vi "TSM SSC DAQmx Configure Digital Edge Start trigger PXI Trig.vi"(0 "DAQ TSM in":T1, 5 "source(PXI_Trig0)":string(combo)="PXI_Trig0", 7 "Edge":i32(ring)=10280 items=["Rising"=10280, "Falling"=10171], 11 "error in (no error)":errorcluster) -> (4 "DAQ TSM Out":T1, 15 "error out":errorcluster)   [LabVIEW 2020]
doc: "Configures the task to start acquiring or generating samples on a rising or falling edge of a digital signal."
uses:
  Pin Map/TSM DAQmx Multi-Task.ctl
  <vilib>/NI_TestStand_SemiconductorModule/NI_TestStand_Semiconductor_Module.lvlibp/PinMap/PinQueryContext/MultiplePinMultipleSessionQueryContext/MultiplePinMultipleSessionQueryContext.lvclass
  Pin Map/SSC DAQmx.ctl
  <vilib>/DAQmx/configure/trigger.llb/DAQmx Start Trigger (Digital Edge).vi
  <resource>/objmgr/daqmx.rc
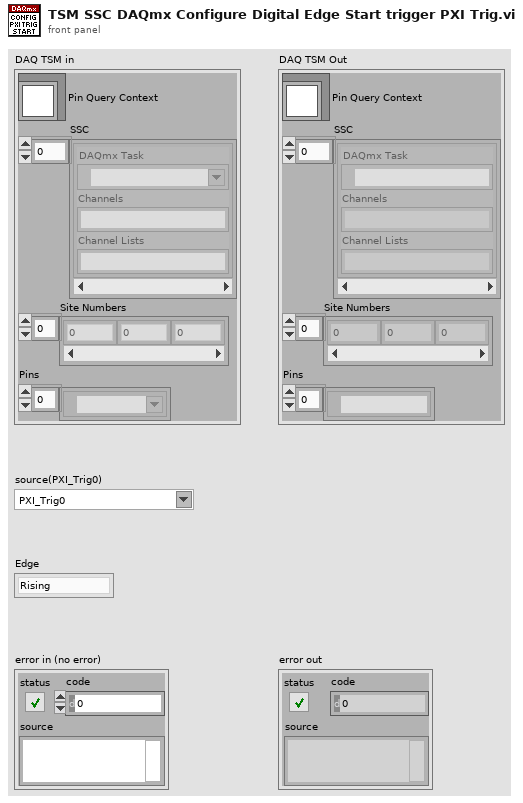
[diagram p1: front panel]
types:
  T1 = typedef "TSM DAQmx Multi-Task.ctl" = cluster{"Pin Query Context":refnum<class "MultiplePinMultipleSessionQueryContext.lvclass">, "SSC":T2[], "Site Numbers":i32[], "Pins":tag[]}
  T2 = typedef "SSC DAQmx.ctl" = cluster{"DAQmx Task ":refnum<k21>, "Channels":string, "Channel Lists":string}
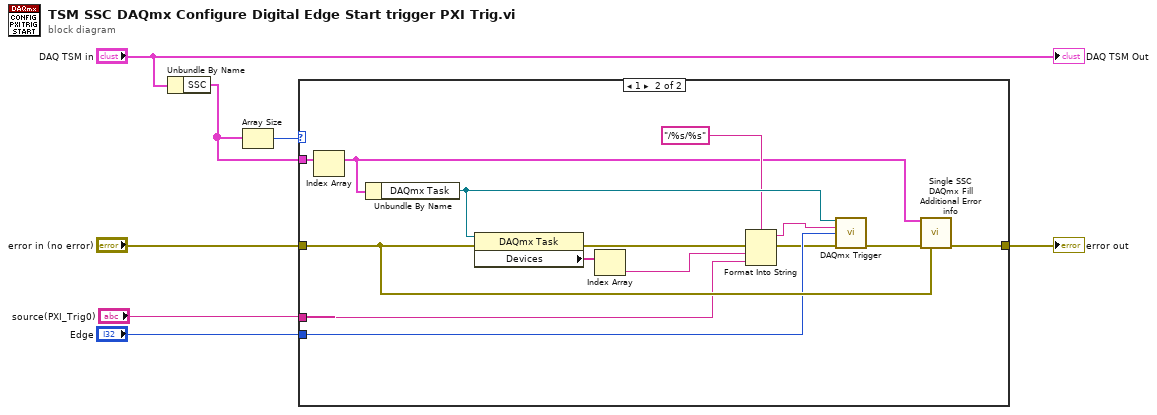
[diagram p0: block diagram]
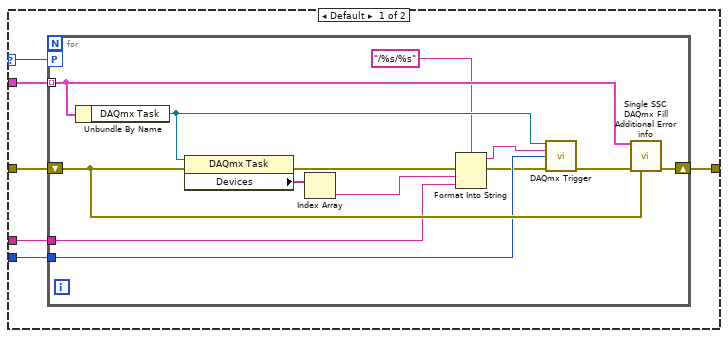
[diagram p2: hidden frame]
diagram:
  n1 = Unbundle By Name("DAQ TSM in") -> ("SSC"=w4:T2[])
  n2 = Array Size(array=w4) -> (size(s)=w6:i32)
  n3 = case shown="1" w6 {
    selector: w6 -> [w11 _]
    tunnel: [w13 w40] -> w2
    tunnel: "error in (no error)" -> [w12 w39]
    tunnel: w4 -> [w10 w38]
    tunnel: "Edge" -> [w9 w37]
    tunnel: "source(PXI_Trig0)" -> [w8 w36]
    frame Default {
      n4 = for {
        tunnel: w10 -> [w25] mode=indexing
        workers-P: w11 -> [_]
        shift-right: [w26] -> w13
        shift-left: w12 -> [w24]
        tunnel: w9 -> [w22]
        tunnel: w8 -> [w14]
        n5 = Unbundle By Name(w25) -> ("DAQmx Task"=w21:refnum<k21>)
        n6 = property class="DAQmx Task"(reference=w21, error in=w24) -> (error out=w20:errorcluster, "Devices"=w17:tag[])  [unwired: 1 out]
        n7 = Index Array(array=w17) -> (element=w16:tag)  [unwired: 1 in]
        n8 = Format Into String(format string="/%s/%s", error in=w20, w16, w14) -> (resulting string=w15:string, error out=w19:errorcluster)  [unwired: 1 in]
        n9 = call-poly <vilib>:"DAQmx Trigger.vi"("task/channels in"=w21, "source"=w15, "edge"=w22, "error in"=w19) -> ("error out"=w23:errorcluster)  [unwired: 10 in, 1 out]
        n10 = call "Single SSC DAQmx Fill Additional Error info.vi"("DAQmx SSC in"=w25, "error in"=w23, "previous error in"=w24) -> ("error out"=w26:errorcluster)  [unwired: 12 in]
      }
    }
    frame 1 {
      n11 = Index Array(array=w38) -> (element=w27:T2)  [unwired: 1 in]
      n12 = Unbundle By Name(w27) -> ("DAQmx Task"=w34:refnum<k21>)
      n13 = property class="DAQmx Task"(reference=w34, error in=w39) -> (error out=w33:errorcluster, "Devices"=w30:tag[])  [unwired: 1 out]
      n14 = Index Array(array=w30) -> (element=w29:tag)  [unwired: 1 in]
      n15 = Format Into String(format string="/%s/%s", error in=w33, w29, w36) -> (resulting string=w28:string, error out=w32:errorcluster)  [unwired: 1 in]
      n16 = call-poly <vilib>:"DAQmx Trigger.vi"("task/channels in"=w34, "source"=w28, "edge"=w37, "error in"=w32) -> ("error out"=w35:errorcluster)  [unwired: 10 in, 1 out]
      n17 = call "Single SSC DAQmx Fill Additional Error info.vi"("DAQmx SSC in"=w27, "error in"=w35, "previous error in"=w39) -> ("error out"=w40:errorcluster)  [unwired: 12 in]
    }
  }
  "error out" <- w2
  "DAQ TSM Out" <- "DAQ TSM in"
